vi "StahlPS_Pbus.ProcCases.vi"(0 "i ref in":refnum<vi>, 1 "selector":string, 2 "Data":T1, 3 "call cluster":T2={"Object"="", "Selector"="", "CallType"=enum."synchronous", "Async Object"="", "Async Selector"="", "Data Descriptor"="", "Data"=[], "Error #"=0, "Expire"=0}, 5 "error in (no error)":errorcluster) -> (14 "i ref out":refnum<vi>, 17 "answer cluster":T2={"Object"="", "Selector"="", "CallType"=enum."synchronous", "Async Object"="", "Async Selector"="", "Data Descriptor"="", "Data"=[], "Error #"=0, "Expire"=0}, 19 "error out":errorcluster)   [LabVIEW 2014, in "StahlPS_Pbus.lvlib"]
doc: "This method is called by a process from within the default case in the event loop. The methods of a class that are linked to events will be called from THIS method. Add your code here."
uses:
  StahlPS_Pbus.lvlib
  CSCore/CSSystem/CoreDefs/CoreDefs.call_type.ctl
  CSCore/BaseProcess/BaseProcess.descriptor string definition.ctl
  CSCore/CSSystem/CoreDefs/CoreDefs.rawDataType.ctl
  CSCore/CSSystem/CoreLib/CoreLib.string 2 byte array.vi
  CSCore/CSSystem/CoreLib/CoreLib.byte array 2 double.vi
  CSCore/CSSystem/CoreLib/CoreLib.byte array 2 int.vi
  CSCore/CSSystem/CoreLib/CoreLib.lvlib
  CSCore/BaseProcess/BaseProcess.lvlib
  CSCore/CAEObj/CAEObj.lvlib
  CSCore/CSApplicationBaseClasses/PSChannelBase/PSChannelBase.lvlib
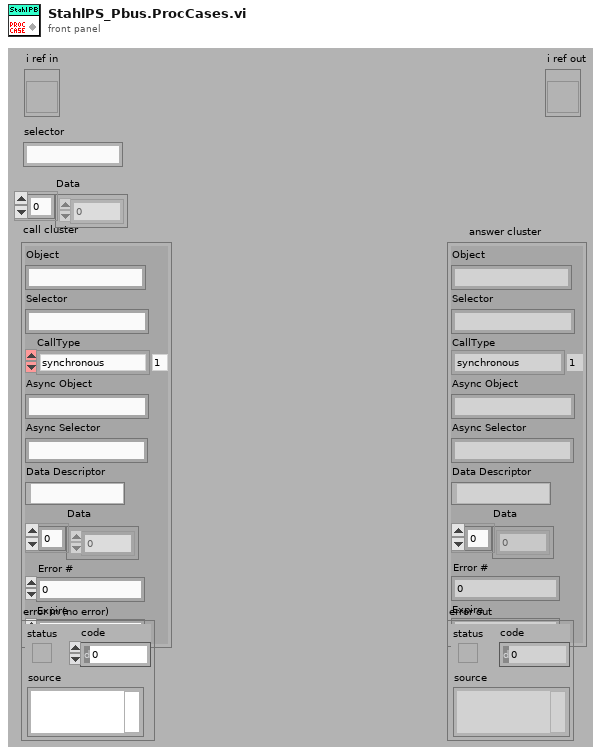
[diagram p1: front panel]
types:
  T1 = typedef "CoreDefs.rawDataType.ctl" = i8[]
  T2 = typedef "CoreDefs.call_type.ctl" = cluster{"Object":string, "Selector":string, "CallType":enum16{"simple", "synchronous", "asynchronous"}, "Async Object":string, "Async Selector":string, "Data Descriptor":T3, "Data":T1, "Error #":i32, "Expire":u32}
  T3 = typedef "BaseProcess.lvlib/BaseProcess.descriptor string definition.ctl" = string
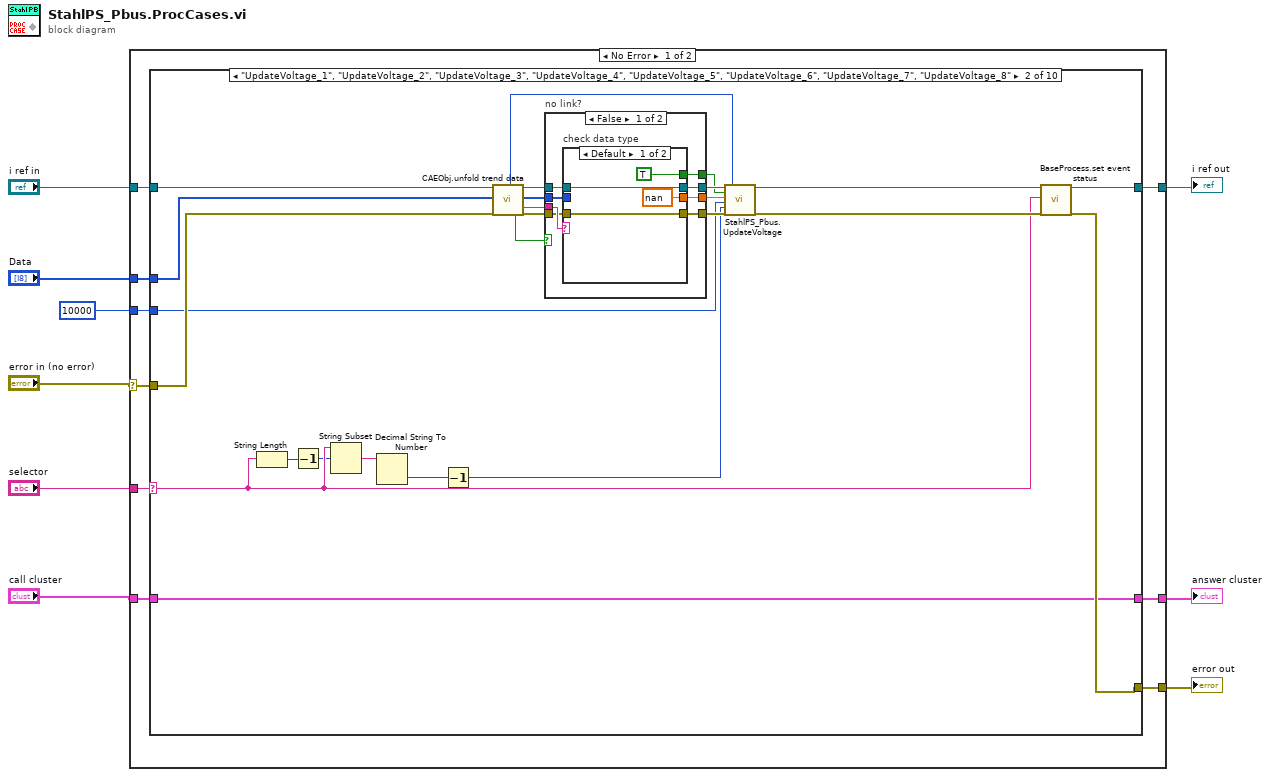
[diagram p0: block diagram]
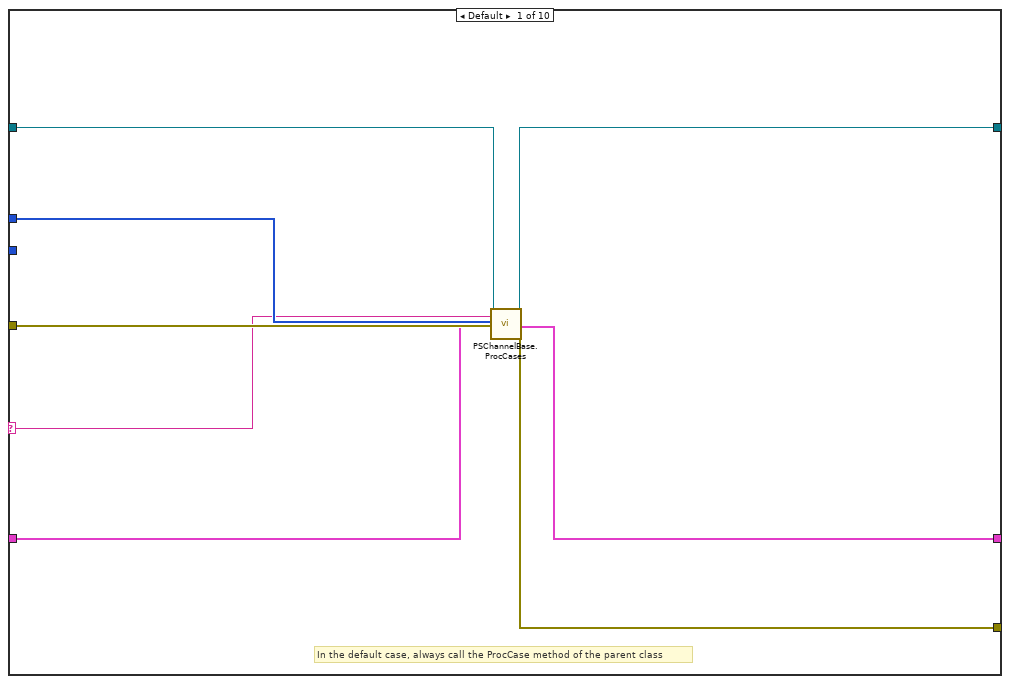
[diagram p2: hidden frame]
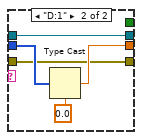
[diagram p3: hidden frame]
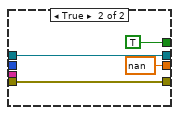
[diagram p4: hidden frame]
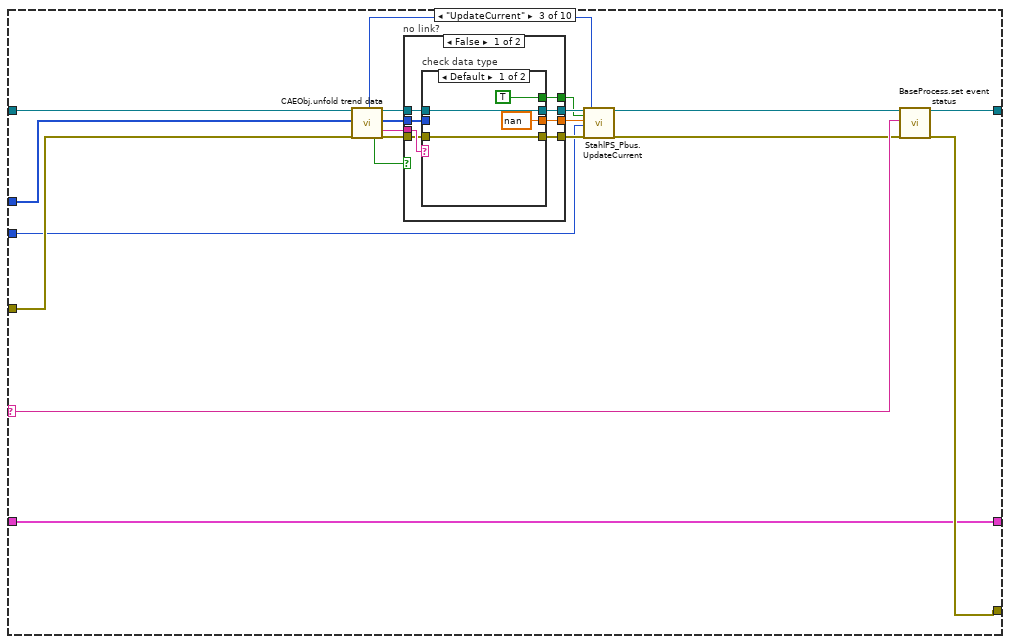
[diagram p5: hidden frame]
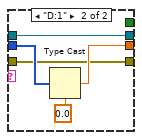
[diagram p6: hidden frame]
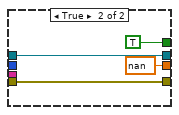
[diagram p7: hidden frame]
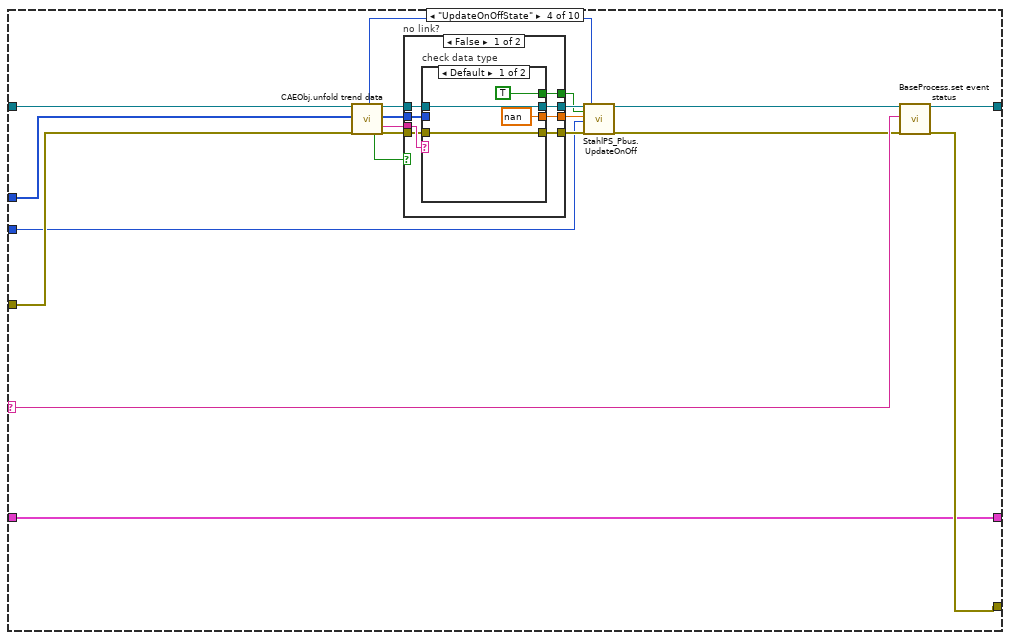
[diagram p8: hidden frame]
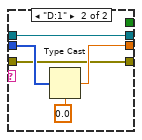
[diagram p9: hidden frame]
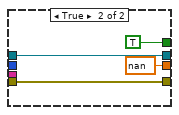
[diagram p10: hidden frame]
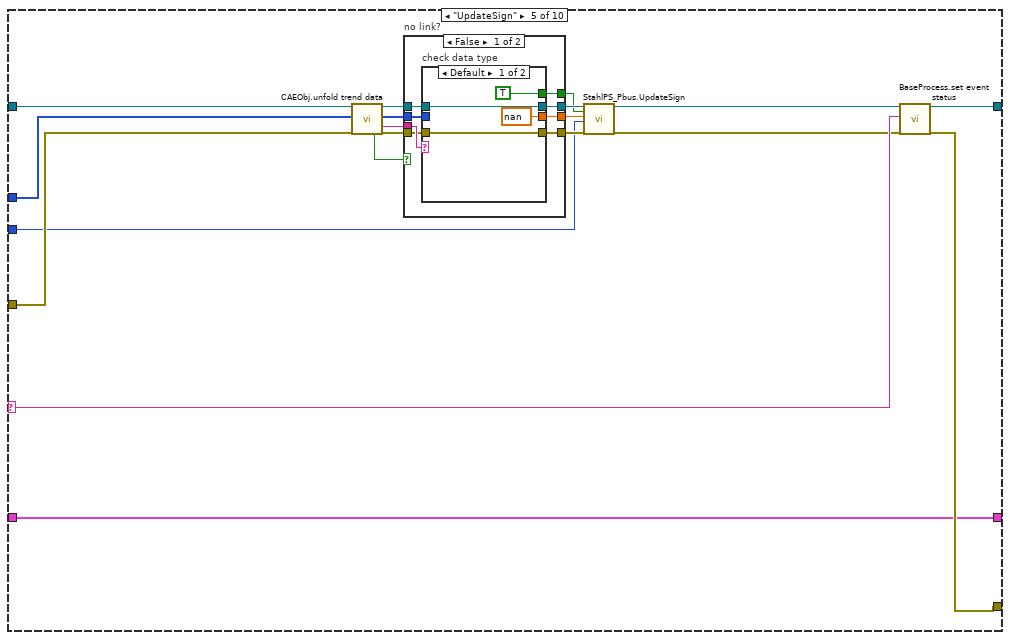
[diagram p11: hidden frame]
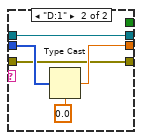
[diagram p12: hidden frame]
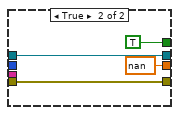
[diagram p13: hidden frame]
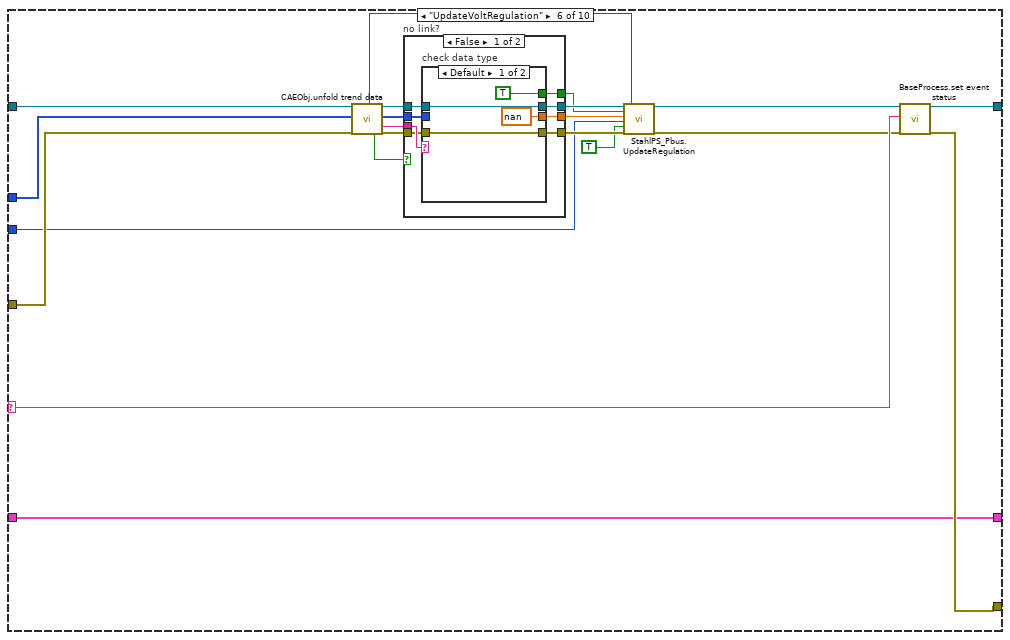
[diagram p14: hidden frame]
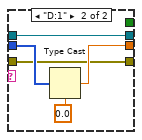
[diagram p15: hidden frame]
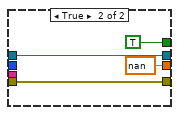
[diagram p16: hidden frame]
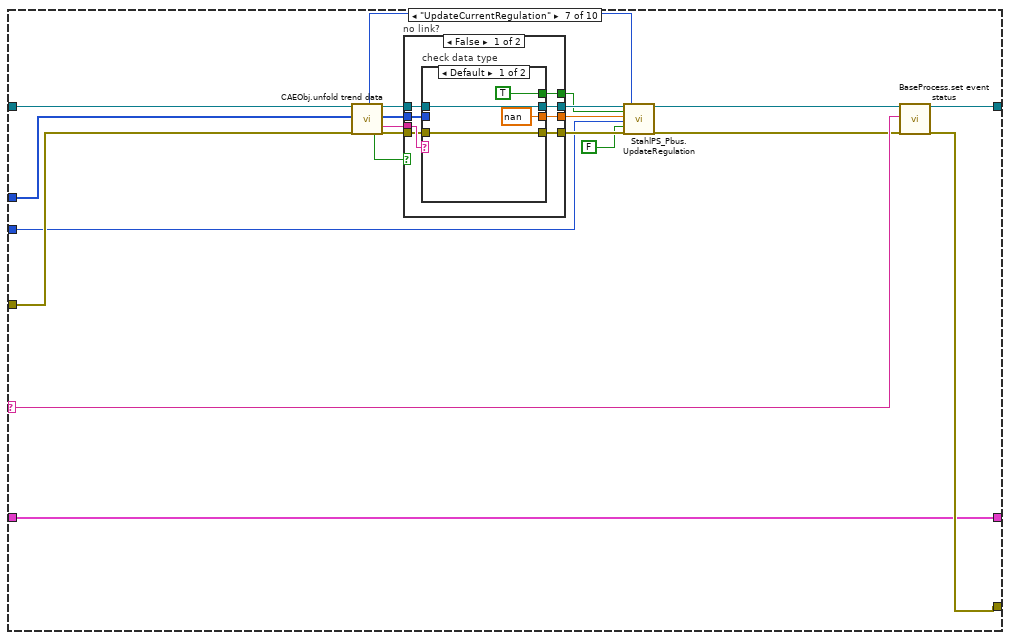
[diagram p17: hidden frame]
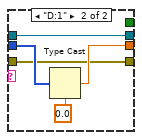
[diagram p18: hidden frame]
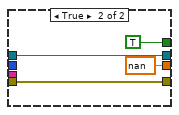
[diagram p19: hidden frame]
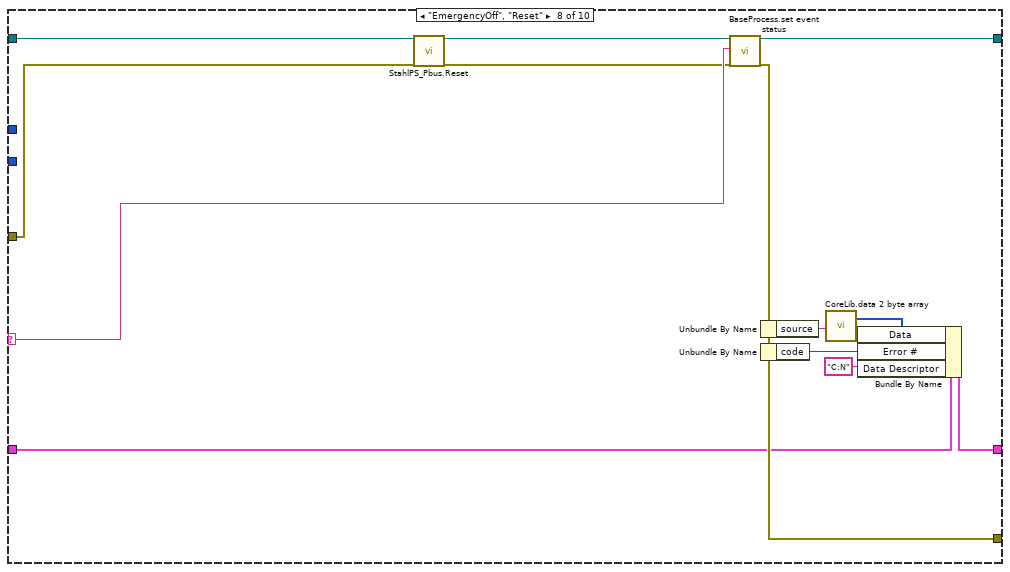
[diagram p20: hidden frame]
diagram:
  n1 = case shown="No Error" "error in (no error)" {
    selector: "error in (no error)" -> [w11 w350]
    tunnel: "selector" -> [w18 _]
    tunnel: [w17 w351] -> w3
    tunnel: "Data" -> [w16 _]
    tunnel: "call cluster" -> [w15 w351]
    tunnel: "i ref in" -> [w14 w352]
    tunnel: [w13 w352] -> w4
    tunnel: [w12 w350] -> w2
    tunnel: 10000 ("ms timeout (100)") -> [w10 _]
    frame No Error {
      n2 = case shown="\"UpdateVoltage_1\", \"UpdateVoltage_2\", \"UpdateVoltage_3\", \"UpdateVoltage_4\", \"UpdateVoltage_5\", \"UpdateVoltage_6\", \"UpdateVoltage_7\", \"UpdateVoltage_8\"" w18 {
        selector: w18 -> [w20 w32 w86 w127 w167 w209 w251 w288 w303 w333]
        tunnel: w16 -> [w21 w46 w87 w128 w168 w210 w252 _ _ _]
        tunnel: w14 -> [w19 w48 w89 w130 w170 w212 w254 w290 w307 w337]
        tunnel: [w26 w50 w91 w132 w172 w214 w256 w291 w308 w338] -> w13
        tunnel: w15 -> [w22 w49 w90 w131 w171 w213 w255 w280 w293 w324]
        tunnel: [w23 w49 w90 w131 w171 w213 w255 w282 w298 w328] -> w17
        tunnel: w11 -> [w25 w47 w88 w129 w169 w211 w253 w279 w292 w323]
        tunnel: [w24 w51 w92 w133 w173 w215 w257 w281 w297 w327] -> w12
        tunnel: w10 -> [_ w33 w73 w114 w155 w197 w239 _ _ _]
        frame Default {
          # "In the default case, always call the ProcCase method of the parent class"
          n3 = call "PSChannelBase.ProcCases.vi"("i ref in"=w19, "selector"=w20, "Data"=w21, "call cluster"=w22, "error in (no error)"=w25) -> ("i ref out"=w26:refnum<vi>, "answer cluster"=w23:T2, "error out"=w24:errorcluster)  [unwired: 12 in]
        }
        frame "UpdateVoltage_1", "UpdateVoltage_2", "UpdateVoltage_3", "UpdateVoltage_4", "UpdateVoltage_5", "UpdateVoltage_6", "UpdateVoltage_7", "UpdateVoltage_8" {
          n4 = String Length(string=w32) -> (length=w31:i32)
          n5 = Decrement(x=w31) -> (x-1=w30:i32)
          n6 = String Subset(string=w32, offset (0)=w30) -> (substring=w29:string)  [unwired: 1 in]
          n7 = Decimal String To Number(string=w29) -> (number=w28:i32)  [unwired: 2 in, 1 out]
          n8 = Decrement(x=w28) -> (x-1=w27:i32)
          n9 = call "CAEObj.unfold trend data.vi"("i ref in"=w48, "raw trend data"=w46, "error in (no error)"=w47) -> ("quality"=w34:i32, "no link"=w41:bool, "i ref out"=w45:refnum<vi>, "data"=w43:i8[], "typeDescriptor"=w42:string, "error out"=w44:errorcluster)  [unwired: 8 in, 3 out]
          n10 = case "no link?" shown="False" w41 {
            tunnel: [w59 w71] -> w40
            tunnel: [w58 w70] -> w39
            tunnel: w43 -> [w57 _]
            tunnel: w45 -> [w56 w71]
            tunnel: w42 -> [w55 _]
            tunnel: w44 -> [w54 w70]
            tunnel: [w53 TRUE ("badValue")] -> w36
            tunnel: [w52 nan] -> w35
            frame False {
              n11 = case "check data type" shown="Default" w55 {
                tunnel: [w61 w64] -> w59
                tunnel: [w62 w65] -> w58
                tunnel: w57 -> [_ w68]
                tunnel: w56 -> [w61 w64]
                tunnel: w54 -> [w62 w65]
                tunnel: [TRUE ("badValue") _] -> w53
                tunnel: [nan w66] -> w52
                frame Default {
                }
                frame "D:1" {
                  n12 = Type Cast(type=0.0, x=w68) -> (*(type *) &x=w66:dbl)
                }
              }
            }
            frame True {
            }
          }
          n13 = call "StahlPS_Pbus.UpdateVoltage.vi"("i ref in"=w40, "badValue"=w36, "moduleValue"=w35, "ms timeout (10000)"=w33, "channelNumber"=w27, "error in (no error)"=w39, "voltageQuality"=w34) -> ("i ref out"=w38:refnum<vi>, "error out"=w37:errorcluster)  [unwired: 10 in, 1 out]
          n14 = call "BaseProcess.set event status.vi"("i ref in"=w38, "EventStatus"=w32, "error in (no error)"=w37) -> ("i ref out"=w50:refnum<vi>, "error out"=w51:errorcluster)  [unwired: 14 in, 1 out]
        }
        frame "UpdateCurrent" {
          n15 = call "CAEObj.unfold trend data.vi"("i ref in"=w89, "raw trend data"=w87, "error in (no error)"=w88) -> ("quality"=w74:i32, "no link"=w81:bool, "i ref out"=w85:refnum<vi>, "data"=w83:i8[], "typeDescriptor"=w82:string, "error out"=w84:errorcluster)  [unwired: 8 in, 3 out]
          n16 = case "no link?" shown="False" w81 {
            tunnel: [w100 w112] -> w80
            tunnel: [w99 w111] -> w79
            tunnel: w83 -> [w98 _]
            tunnel: w85 -> [w97 w112]
            tunnel: w82 -> [w96 _]
            tunnel: w84 -> [w95 w111]
            tunnel: [w94 TRUE ("badValue")] -> w76
            tunnel: [w93 nan] -> w75
            frame False {
              n17 = case "check data type" shown="Default" w96 {
                tunnel: [w102 w105] -> w100
                tunnel: [w103 w106] -> w99
                tunnel: w98 -> [_ w109]
                tunnel: w97 -> [w102 w105]
                tunnel: w95 -> [w103 w106]
                tunnel: [TRUE ("badValue") _] -> w94
                tunnel: [nan w107] -> w93
                frame Default {
                }
                frame "D:1" {
                  n18 = Type Cast(type=0.0, x=w109) -> (*(type *) &x=w107:dbl)
                }
              }
            }
            frame True {
            }
          }
          n19 = call "StahlPS_Pbus.UpdateCurrent.vi"("i ref in"=w80, "badValue"=w76, "moduleValue"=w75, "ms timeout (10000)"=w73, "error in (no error)"=w79, "quality"=w74) -> ("i ref out"=w78:refnum<vi>, "error out"=w77:errorcluster)  [unwired: 11 in, 1 out]
          n20 = call "BaseProcess.set event status.vi"("i ref in"=w78, "EventStatus"=w86, "error in (no error)"=w77) -> ("i ref out"=w91:refnum<vi>, "error out"=w92:errorcluster)  [unwired: 14 in, 1 out]
        }
        frame "UpdateOnOffState" {
          n21 = call "CAEObj.unfold trend data.vi"("i ref in"=w130, "raw trend data"=w128, "error in (no error)"=w129) -> ("quality"=w115:i32, "no link"=w122:bool, "i ref out"=w126:refnum<vi>, "data"=w124:i8[], "typeDescriptor"=w123:string, "error out"=w125:errorcluster)  [unwired: 8 in, 3 out]
          n22 = case "no link?" shown="False" w122 {
            tunnel: [w141 w153] -> w121
            tunnel: [w140 w152] -> w120
            tunnel: w124 -> [w139 _]
            tunnel: w126 -> [w138 w153]
            tunnel: w123 -> [w137 _]
            tunnel: w125 -> [w136 w152]
            tunnel: [w135 TRUE ("badValue")] -> w117
            tunnel: [w134 nan] -> w116
            frame False {
              n23 = case "check data type" shown="Default" w137 {
                tunnel: [w143 w146] -> w141
                tunnel: [w144 w147] -> w140
                tunnel: w139 -> [_ w150]
                tunnel: w138 -> [w143 w146]
                tunnel: w136 -> [w144 w147]
                tunnel: [TRUE ("badValue") _] -> w135
                tunnel: [nan w148] -> w134
                frame Default {
                }
                frame "D:1" {
                  n24 = Type Cast(type=0.0, x=w150) -> (*(type *) &x=w148:dbl)
                }
              }
            }
            frame True {
            }
          }
          n25 = call "StahlPS_Pbus.UpdateOnOff.vi"("i ref in"=w121, "badValue"=w117, "moduleValue"=w116, "ms timeout (10000)"=w114, "error in (no error)"=w120, "onOffQuality"=w115) -> ("i ref out"=w119:refnum<vi>, "error out"=w118:errorcluster)  [unwired: 11 in, 1 out]
          n26 = call "BaseProcess.set event status.vi"("i ref in"=w119, "EventStatus"=w127, "error in (no error)"=w118) -> ("i ref out"=w132:refnum<vi>, "error out"=w133:errorcluster)  [unwired: 14 in, 1 out]
        }
        frame "UpdateSign" {
          n27 = call "CAEObj.unfold trend data.vi"("i ref in"=w170, "raw trend data"=w168, "error in (no error)"=w169) -> ("no link"=w162:bool, "i ref out"=w166:refnum<vi>, "data"=w164:i8[], "typeDescriptor"=w163:string, "error out"=w165:errorcluster)  [unwired: 8 in, 4 out]
          n28 = case "no link?" shown="False" w162 {
            tunnel: [w181 w193] -> w161
            tunnel: [w180 w192] -> w160
            tunnel: w164 -> [w179 _]
            tunnel: w166 -> [w178 w193]
            tunnel: w163 -> [w177 _]
            tunnel: w165 -> [w176 w192]
            tunnel: [w175 TRUE ("badValue")] -> w157
            tunnel: [w174 nan] -> w156
            frame False {
              n29 = case "check data type" shown="Default" w177 {
                tunnel: [w183 w186] -> w181
                tunnel: [w184 w187] -> w180
                tunnel: w179 -> [_ w190]
                tunnel: w178 -> [w183 w186]
                tunnel: w176 -> [w184 w187]
                tunnel: [TRUE ("badValue") _] -> w175
                tunnel: [nan w188] -> w174
                frame Default {
                }
                frame "D:1" {
                  n30 = Type Cast(type=0.0, x=w190) -> (*(type *) &x=w188:dbl)
                }
              }
            }
            frame True {
            }
          }
          n31 = call "StahlPS_Pbus.UpdateSign.vi"("i ref in"=w161, "badValue"=w157, "moduleValue"=w156, "ms timeout (10000)"=w155, "error in (no error)"=w160) -> ("i ref out"=w159:refnum<vi>, "error out"=w158:errorcluster)  [unwired: 12 in, 1 out]
          n32 = call "BaseProcess.set event status.vi"("i ref in"=w159, "EventStatus"=w167, "error in (no error)"=w158) -> ("i ref out"=w172:refnum<vi>, "error out"=w173:errorcluster)  [unwired: 14 in, 1 out]
        }
        frame "UpdateVoltRegulation" {
          n33 = call "CAEObj.unfold trend data.vi"("i ref in"=w212, "raw trend data"=w210, "error in (no error)"=w211) -> ("quality"=w196:i32, "no link"=w204:bool, "i ref out"=w208:refnum<vi>, "data"=w206:i8[], "typeDescriptor"=w205:string, "error out"=w207:errorcluster)  [unwired: 8 in, 3 out]
          n34 = case "no link?" shown="False" w204 {
            tunnel: [w223 w235] -> w203
            tunnel: [w222 w234] -> w202
            tunnel: w206 -> [w221 _]
            tunnel: w208 -> [w220 w235]
            tunnel: w205 -> [w219 _]
            tunnel: w207 -> [w218 w234]
            tunnel: [w217 TRUE ("badValue")] -> w199
            tunnel: [w216 nan] -> w198
            frame False {
              n35 = case "check data type" shown="Default" w219 {
                tunnel: [w225 w228] -> w223
                tunnel: [w226 w229] -> w222
                tunnel: w221 -> [_ w232]
                tunnel: w220 -> [w225 w228]
                tunnel: w218 -> [w226 w229]
                tunnel: [TRUE ("badValue") _] -> w217
                tunnel: [nan w230] -> w216
                frame Default {
                }
                frame "D:1" {
                  n36 = Type Cast(type=0.0, x=w232) -> (*(type *) &x=w230:dbl)
                }
              }
            }
            frame True {
            }
          }
          n37 = call "StahlPS_Pbus.UpdateRegulation.vi"("i ref in"=w203, "badValue"=w199, "moduleValue"=w198, "ms timeout (10000)"=w197, "voltageRegulation"=TRUE, "error in (no error)"=w202, "valueQuality"=w196) -> ("i ref out"=w201:refnum<vi>, "error out"=w200:errorcluster)  [unwired: 10 in, 1 out]
          n38 = call "BaseProcess.set event status.vi"("i ref in"=w201, "EventStatus"=w209, "error in (no error)"=w200) -> ("i ref out"=w214:refnum<vi>, "error out"=w215:errorcluster)  [unwired: 14 in, 1 out]
        }
        frame "UpdateCurrentRegulation" {
          n39 = call "CAEObj.unfold trend data.vi"("i ref in"=w254, "raw trend data"=w252, "error in (no error)"=w253) -> ("quality"=w238:i32, "no link"=w246:bool, "i ref out"=w250:refnum<vi>, "data"=w248:i8[], "typeDescriptor"=w247:string, "error out"=w249:errorcluster)  [unwired: 8 in, 3 out]
          n40 = case "no link?" shown="False" w246 {
            tunnel: [w265 w277] -> w245
            tunnel: [w264 w276] -> w244
            tunnel: w248 -> [w263 _]
            tunnel: w250 -> [w262 w277]
            tunnel: w247 -> [w261 _]
            tunnel: w249 -> [w260 w276]
            tunnel: [w259 TRUE ("badValue")] -> w241
            tunnel: [w258 nan] -> w240
            frame False {
              n41 = case "check data type" shown="Default" w261 {
                tunnel: [w267 w270] -> w265
                tunnel: [w268 w271] -> w264
                tunnel: w263 -> [_ w274]
                tunnel: w262 -> [w267 w270]
                tunnel: w260 -> [w268 w271]
                tunnel: [TRUE ("badValue") _] -> w259
                tunnel: [nan w272] -> w258
                frame Default {
                }
                frame "D:1" {
                  n42 = Type Cast(type=0.0, x=w274) -> (*(type *) &x=w272:dbl)
                }
              }
            }
            frame True {
            }
          }
          n43 = call "StahlPS_Pbus.UpdateRegulation.vi"("i ref in"=w245, "badValue"=w241, "moduleValue"=w240, "ms timeout (10000)"=w239, "voltageRegulation"=FALSE, "error in (no error)"=w244, "valueQuality"=w238) -> ("i ref out"=w243:refnum<vi>, "error out"=w242:errorcluster)  [unwired: 10 in, 1 out]
          n44 = call "BaseProcess.set event status.vi"("i ref in"=w243, "EventStatus"=w251, "error in (no error)"=w242) -> ("i ref out"=w256:refnum<vi>, "error out"=w257:errorcluster)  [unwired: 14 in, 1 out]
        }
        frame "EmergencyOff", "Reset" {
          n45 = call "StahlPS_Pbus.Reset.vi"("i ref in"=w290, "error in (no error)"=w279) -> ("i ref out"=w289:refnum<vi>, "error out (no error)"=w287:errorcluster)  [unwired: 16 in]
          n46 = call "BaseProcess.set event status.vi"("i ref in"=w289, "EventStatus"=w288, "error in (no error)"=w287) -> ("i ref out"=w291:refnum<vi>, "error out"=w281:errorcluster)  [unwired: 14 in, 1 out]
          n47 = Unbundle By Name(w281) -> ("source"=w283:string)
          n48 = Unbundle By Name(w281) -> ("code"=w286:i32)
          n49 = call-poly "CoreLib.data 2 byte array.vi"("string"=w283) -> ("byteArray out"=w285:T1)  [unwired: 18 in]
          n50 = Bundle By Name(cluster=w280, "Data"=w285, "Error #"=w286, "Data Descriptor"="C:N") -> (w282:T2)
        }
        frame "SetVoltage" {
          n51 = Unbundle By Name(w293) -> ("Data"=w296:T1)
          n52 = call-poly "CoreLib.byte array 2 data.vi"("byteArray"=w296) -> ("d64"=w294:dbl, "error out"=w295:errorcluster)  [unwired: 16 in, 1 out]
          n53 = case shown="No Error" w295 {
            selector: w295 -> [_ w318]
            tunnel: w303 -> [w311 w317]
            tunnel: [w311 w317] -> w305
            tunnel: [w312 w316] -> w304
            tunnel: w307 -> [w314 w315]
            tunnel: [w313 w315] -> w306
            tunnel: w294 -> [w310 _]
            tunnel: w292 -> [w309 _]
            frame No Error {
              n54 = call "StahlPS_Pbus.SetVoltage.vi"("i ref in"=w314, "value"=w310, "error in (no error)"=w309) -> ("i ref out"=w313:refnum<vi>, "error out (no error)"=w312:errorcluster)  [unwired: 15 in]
            }
            frame Error {
              n55 = call "CoreLib.set data type mismatch.vi"("error in (no error)"=w318, "error source"=w317) -> ("error out"=w316:errorcluster)  [unwired: 17 in]
            }
          }
          n56 = call "BaseProcess.set event status.vi"("i ref in"=w306, "EventStatus"=w305, "error in (no error)"=w304) -> ("i ref out"=w308:refnum<vi>, "error out"=w297:errorcluster)  [unwired: 14 in, 1 out]
          n57 = Unbundle By Name(w297) -> ("source"=w299:string)
          n58 = Unbundle By Name(w297) -> ("code"=w302:i32)
          n59 = call-poly "CoreLib.data 2 byte array.vi"("string"=w299) -> ("byteArray out"=w301:T1)  [unwired: 18 in]
          n60 = Bundle By Name(cluster=w293, "Data"=w301, "Error #"=w302, "Data Descriptor"="C:N") -> (w298:T2)
        }
        frame "SetChannelVoltage" {
          n61 = Unbundle By Name(w324) -> ("Data"=w322:T1)
          n62 = call-poly "CoreLib.byte array 2 data.vi"("byteArray"=w322) -> ("byteArray out"=w320:T1, "i32"=w319:i32, "error out"=w321:errorcluster)  [unwired: 16 in]
          n63 = call-poly "CoreLib.byte array 2 data.vi"("byteArray"=w320, "error in (no error)"=w321) -> ("d64"=w325:dbl, "error out"=w326:errorcluster)  [unwired: 15 in, 1 out]
          n64 = case shown="No Error" w326 {
            selector: w326 -> [_ w349]
            tunnel: w333 -> [w342 w348]
            tunnel: [w342 w348] -> w335
            tunnel: [w343 w347] -> w334
            tunnel: w337 -> [w345 w346]
            tunnel: [w344 w346] -> w336
            tunnel: w325 -> [w341 _]
            tunnel: w323 -> [w340 _]
            tunnel: w319 -> [w339 _]
            frame No Error {
              n65 = call "StahlPS_Pbus.SetVoltage.vi"("i ref in"=w345, "value"=w341, "error in (no error)"=w340, "channelIndex"=w339) -> ("i ref out"=w344:refnum<vi>, "error out (no error)"=w343:errorcluster)  [unwired: 14 in]
            }
            frame Error {
              n66 = call "CoreLib.set data type mismatch.vi"("error in (no error)"=w349, "error source"=w348) -> ("error out"=w347:errorcluster)  [unwired: 17 in]
            }
          }
          n67 = call "BaseProcess.set event status.vi"("i ref in"=w336, "EventStatus"=w335, "error in (no error)"=w334) -> ("i ref out"=w338:refnum<vi>, "error out"=w327:errorcluster)  [unwired: 14 in, 1 out]
          n68 = Unbundle By Name(w327) -> ("source"=w329:string)
          n69 = Unbundle By Name(w327) -> ("code"=w332:i32)
          n70 = call-poly "CoreLib.data 2 byte array.vi"("string"=w329) -> ("byteArray out"=w331:T1)  [unwired: 18 in]
          n71 = Bundle By Name(cluster=w324, "Data"=w331, "Error #"=w332, "Data Descriptor"="C:N") -> (w328:T2)
        }
      }
    }
    frame Error {
    }
  }
  "answer cluster" <- w3
  "i ref out" <- w4
  "error out" <- w2
